vi "TCam_WellCalculater.vi"(6 "DrawTempOverlay":bool, 8 "Well Pos":T2[](array[typedef]) {"Y" format="%.2f"; "X" format="%.2f"}, 9 "Pixels":cluster{"X":i32, "Y":i32}[][](array[cluster]), 10 "Image in":T1, 11 "index":i32) -> (1 "Individual Pixels":dbl[](array[numeric]), 2 "Image Out":T1, 3 "mean":dbl format="%0.2f")   [LabVIEW 2024]
uses:
  <vilib>/vision/Image Controls.llb/IMAQ Image.ctl
  <vilib>/Analysis/baseanly.llb/Mean (DBL).vi
  <vilib>/vision/NI_Vision_Development_Module.lvlib
  <vilib>/Analysis/NI_AALBase.lvlib
  <vilib>/Utility/file.llb/Write Delimited Spreadsheet (DBL).vi
panel:
  in  "name or relative path":path
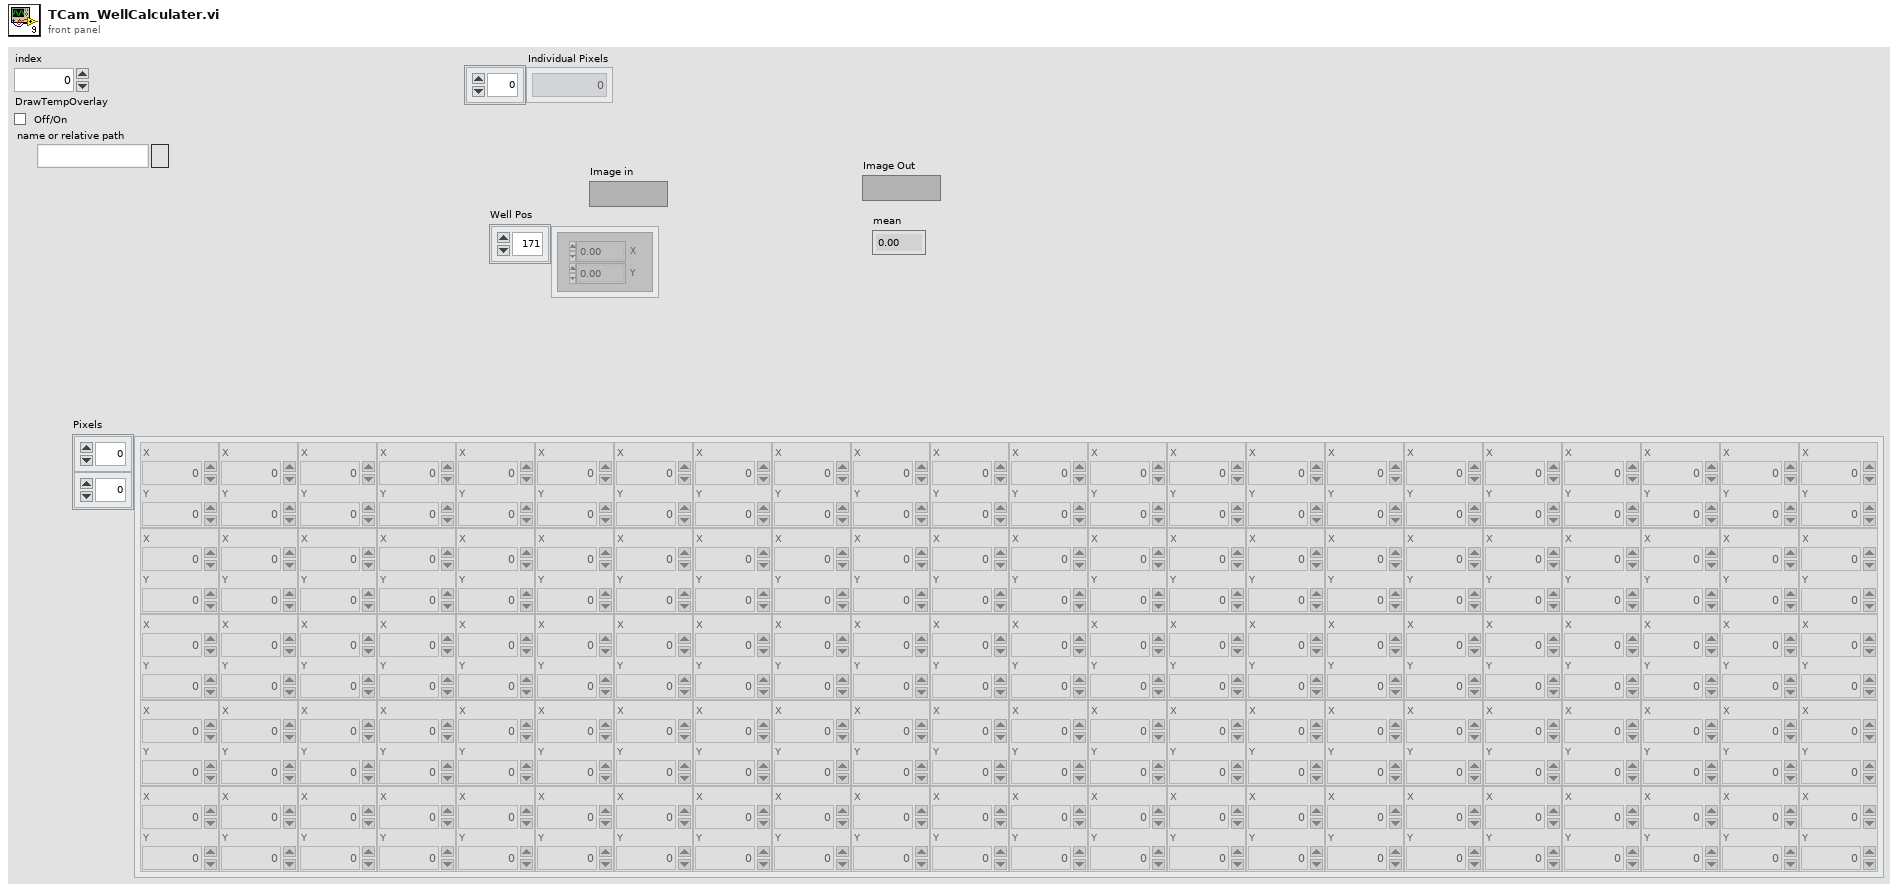
[diagram p1: front panel]
types:
  T1 = typedef "IMAQ Image.ctl" = refnum<image>
  T2 = typedef "IMAQ Point" = cluster{"X":sgl, "Y":sgl}
  T3 = cluster{"Desired Font (Application)":enum16{"User-specified Font", "Application Font", "System Font", "Dialog Font"}, "[User-specified Font]":cluster{"Font Name":string, "Size":i16, "Strikeout?":bool, "Italic?":bool, "Underline?":bool, "Outline?":bool, "Shadow?":bool, "Bold?":bool, "Rotation Angle":dbl}, "Horizontal Alignment":i16, "Vertical Alignment":i16}
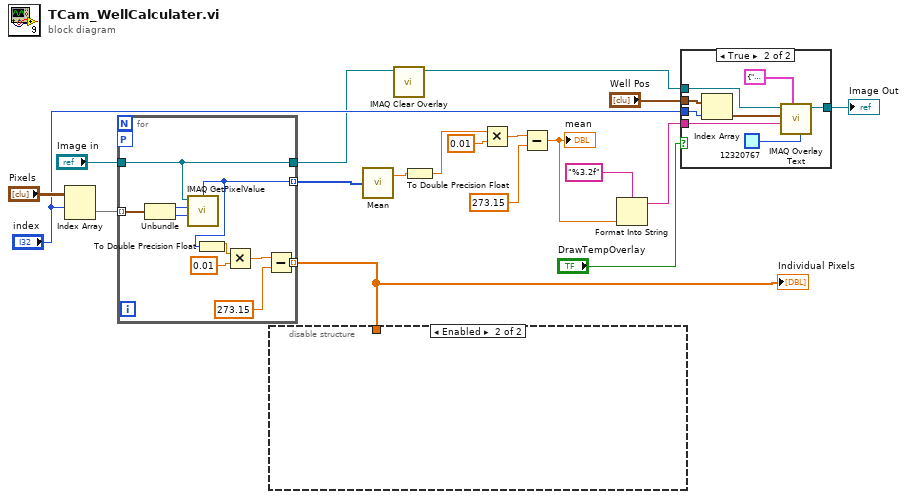
[diagram p0: block diagram]
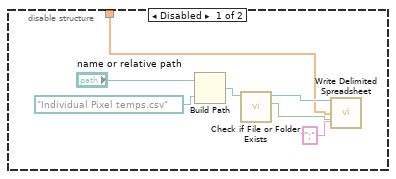
[diagram p2: hidden frame]
diagram:
  n1 = Index Array(array="Pixels", index (row)="index") -> (element=w14:cluster{"X":i32, "Y":i32}[])  [unwired: 1 in]
  n2 = for {
    tunnel: "Image in" -> [w26]
    tunnel: w14 -> [w29] mode=indexing
    tunnel: [w25] -> w2 mode=indexing
    tunnel: [w26] -> w11
    workers-P: _ -> [_]
    tunnel: [w20] -> w1 mode=indexing
    n3 = Unbundle(w29) -> ("X"=w28:i32, "Y"=w27:i32)
    n4 = call "IMAQ GetPixelValue"("Image"=w26, "X Coordinate"=w28, "Y Coordinate"=w27) -> ("Pixel Value (U16)"=w25:u16)  [unwired: 3 in, 4 out]
    n5 = To Double Precision Float(number=w25) -> (double precision float=w21:dbl)
    n6 = Multiply(x=w21, y=0.01) -> (x*y=w23:dbl)
    n7 = Subtract(x=w23, y=273.15) -> (x-y=w20:dbl)
  }
  "Individual Pixels" <- w1
  n8 = disable-structure shown="Enabled" {
    disable-tunnel: w1 -> [w30 _]
    frame Disabled {
      n9 = Build Path(base path="name or relative path", name or relative path=path "Individual Pixel temps.csv") -> (appended path=w34:path)
      n10 = call <vilib>:"Check if File or Folder Exists.vi"("path"=w34) -> ("file or folder exists?"=w32:bool, "dup path"=w33:path)  [unwired: 8 in, 1 out]
      n11 = call-poly <vilib>:"Write Delimited Spreadsheet.vi"("file path (dialog if empty)"=w33, "1D data"=w30, "append to file? (new file:F)"=w32, "delimiter (\\t)"=";" ("delimiter (\\t)")) -> ()  [unwired: 10 in, 2 out]
    }
    frame Enabled {
    }
  }
  n12 = call-poly <vilib>:"Mean.vi"("X"=w2) -> ("mean"=w5:dbl)  [unwired: 1 out]
  n13 = call "IMAQ Clear Overlay"("Image"=w11) -> ("Image Out"=w10:T1)  [unwired: 9 in, 1 out]
  n14 = To Double Precision Float(number=w5) -> (double precision float=w7:dbl)
  n15 = Multiply(x=w7, y=0.01) -> (x*y=w8:dbl)
  n16 = Subtract(x=w8, y=273.15) -> (x-y=w4:dbl)
  "mean" <- w4
  n17 = Format Into String(format string="%3.2f", w4) -> (resulting string=w12:string)  [unwired: 2 in, 1 out]
  n18 = case shown="True" "DrawTempOverlay" {
    tunnel: [w37 w45] -> w18
    tunnel: "Well Pos" -> [_ w44]
    tunnel: "index" -> [_ w42]
    tunnel: w12 -> [_ w40]
    tunnel: w10 -> [w37 w38]
    frame False {
    }
    frame True {
      n19 = Index Array(array=w44, index=w42) -> (element=w43:T2)
      n20 = call "IMAQ Overlay Text"("BG Color (Transparent)"=u32 12320767, "Font, Size & Style"=T3 {"Desired Font (Application)"=enum."Application Font", "[User-specified Font]"={"Font Name"="", "Size"=6, "Strikeout?"=FALSE, "Italic?"=FALSE, "Underline?"=FALSE, "Outline?"=FALSE, "Shadow?"=FALSE, "Bold?"=FALSE, "Rotation Angle"=0.0}, "Horizontal Alignment"=1, "Vertical Alignment"=0}, "String"=w40, "Origin"=w43, "Image"=w38) -> ("Image Out"=w45:T1)  [unwired: 5 in, 1 out]
    }
  }
  "Image Out" <- w18
